vi "Read Wheel State.vi"(8 "error in (no error)":errorcluster, 10 "wheel state in":T1, 11 "wheel in":refnum<class "NI_Robotics_Wheel.lvclass">) -> (0 "error out":errorcluster, 2 "wheel state out":T1, 3 "wheel out":refnum<class "NI_Robotics_Wheel.lvclass">)   [LabVIEW 2017, in "NI_Robotics_Wheel.lvclass"]
uses:
  <vilib>/robotics/Steering/Wheel/NI_Robotics_Wheel.lvclass
  <vilib>/robotics/Steering/Wheel/Wheel State.ctl
  <vilib>/robotics/Steering/Wheel/NI_Robotics_Wheel.lvclass/NI_Robotics_Wheel.ctl
  <vilib>/robotics/Actuation/Motor Communication/Get Motor Velocity State.vi
  <vilib>/robotics/Actuation/Motor Communication/Check if Valid.vi
  <vilib>/robotics/Utilities/Generate Error.vi
  <vilib>/robotics/Actuation/Motor Communication/NI_Robotics_Motor Communication.lvclass
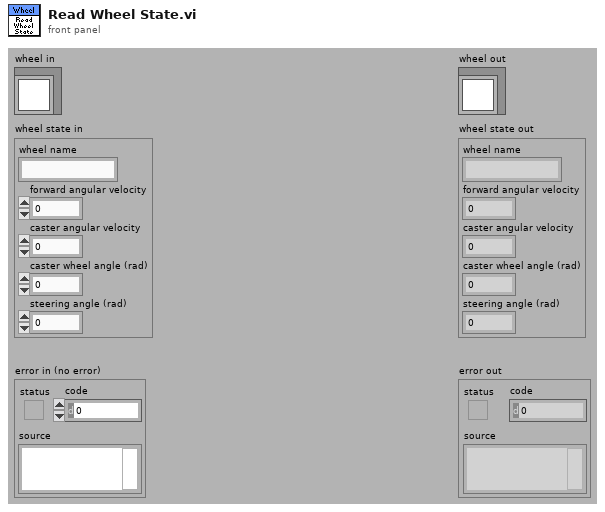
[diagram p1: front panel]
types:
  T1 = typedef "NI_Robotics_Wheel.lvclass/Wheel State.ctl" = cluster{"wheel name":string, "forward angular velocity":dbl, "caster angular velocity":dbl, "caster wheel angle (rad)":dbl, "steering angle (rad)":dbl}
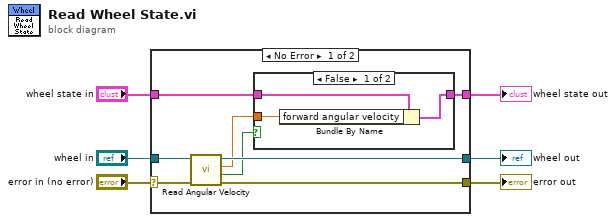
[diagram p0: block diagram]
diagram:
  n1 = case shown="No Error" "error in (no error)" {
    selector: "error in (no error)" -> [w12 w21]
    tunnel: [w11 w21] -> w5
    tunnel: [w13 w20] -> w3
    tunnel: "wheel in" -> [w14 w20]
    tunnel: [w9 w19] -> w2
    tunnel: "wheel state in" -> [w8 w19]
    frame No Error {
      n2 = call <vilib>:"Read Angular Velocity.vi"("error in (no error)"=w12, "wheel in"=w14) -> ("error out"=w11:errorcluster, "failed"=w7:bool, "forward angular velocity"=w10:dbl, "wheel out"=w13:refnum<class "NI_Robotics_Wheel.lvclass">)  [unwired: 6 in]
      n3 = case shown="False" w7 {
        tunnel: w10 -> [w17 _]
        tunnel: [w16 w18] -> w9
        tunnel: w8 -> [w15 w18]
        frame False {
          n4 = Bundle By Name(cluster=w15, "forward angular velocity"=w17) -> (w16:T1)
        }
        frame True {
        }
      }
    }
    frame Error {
    }
  }
  "error out" <- w5
  "wheel out" <- w3
  "wheel state out" <- w2
